vi "Read Intake Current.vi"(8 "Current":dbl, 9 "Proposed Power":dbl, 10 "Max Current":dbl, 11 "Current Trip Delay":dbl) -> (0 "Forward Tripped":bool, 1 "Backward Tripped":bool, 2 "Intake Current Trip State":T1, 3 "Actual Power":dbl, 4 "Current Over Max Current?":bool, 5 "Tripped?":bool)   [LabVIEW 2016]
uses:
  Common Code/Intake Trip States.ctl
  Common Code/Utilities/TimeManager.vi
  Common Code/Utilities/Change Detect.vi
  Common Code/Utilities/Change Detect Boolean.vi
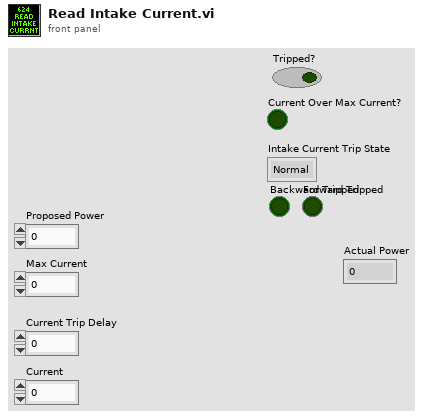
[diagram p1: front panel]
types:
  T1 = typedef "Intake Trip States.ctl" = enum16{"Normal", "Backward Tripped", "Forward Tripped"}
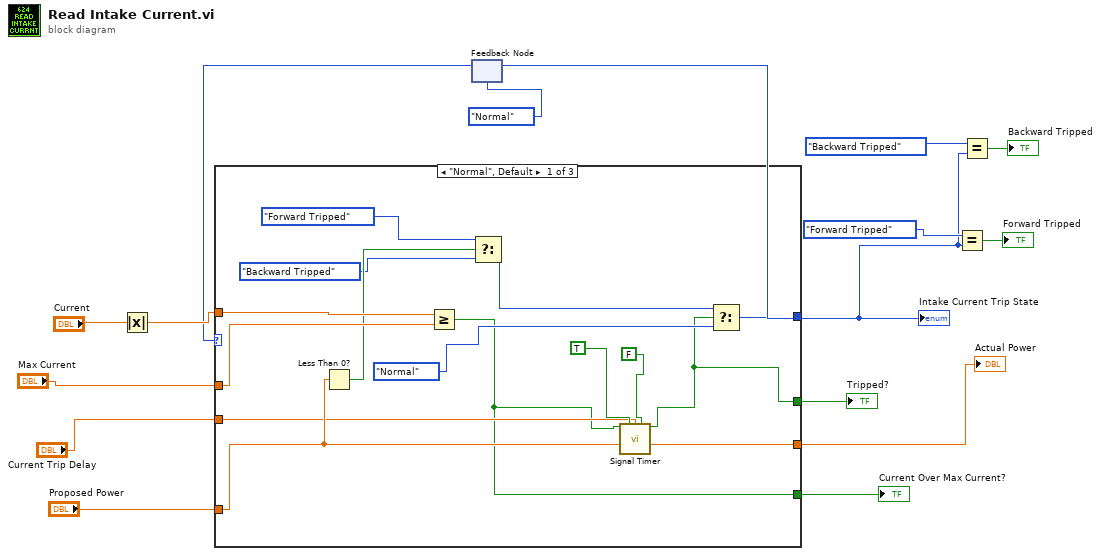
[diagram p0: block diagram]
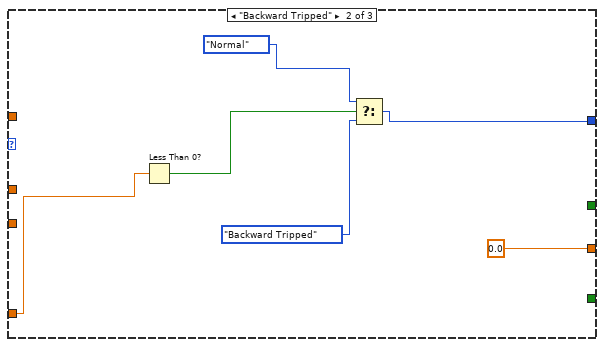
[diagram p2: hidden frame]
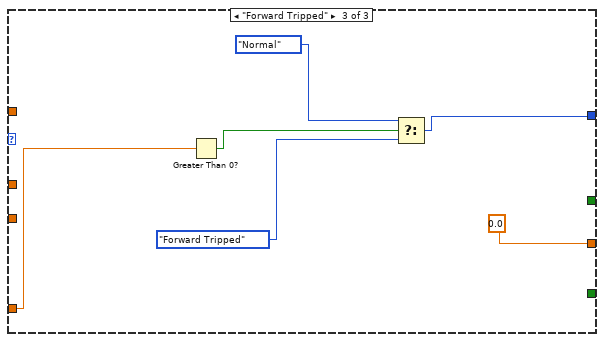
[diagram p3: hidden frame]
diagram:
  n1 = Absolute Value(x="Current") -> (abs(x)=w12:dbl)
  n2 = feedback #1(Intake_Trip_States."Normal" ("Intake Current Trip States")) -> (w3:T1)
  n3 = case shown="\"Normal\", Default" w3 {
    tunnel: "Proposed Power" -> [w25 w30 w40]
    tunnel: [w25 0.0 0.0] -> w15
    tunnel: "Max Current" -> [w28 _ _]
    tunnel: w12 -> [w29 _ _]
    tunnel: [w26 w35 w41] -> w4
    tunnel: "Current Trip Delay" -> [w19 _ _]
    tunnel: [w17 _ _] -> w2
    tunnel: [w16 _ _] -> w1
    frame "Normal", Default {
      n4 = Less Than 0?(x=w25) -> (x < 0?=w24:bool)
      n5 = Greater Or Equal?(x=w29, y=w28) -> (x >= y?=w16:bool)
      n6 = Select(t=Intake_Trip_States."Forward Tripped" ("Intake Current Trip States"), s=w24, f=Intake_Trip_States."Backward Tripped" ("Intake Current Trip States")) -> (s? t:f=w27:T1)
      n7 = call "Signal Timer.vi"("Input"=w16, "Edge"=TRUE, "Interval"=w19, "Pull"=FALSE) -> ("Filtered Output"=w17:bool)  [unwired: 11 in]
      n8 = Select(t=w27, s=w17, f=Intake_Trip_States."Normal" ("Intake Current Trip States")) -> (s? t:f=w26:T1)
    }
    frame "Backward Tripped" {
      n9 = Less Than 0?(x=w30) -> (x < 0?=w31:bool)
      n10 = Select(t=Intake_Trip_States."Normal" ("Intake Current Trip States"), s=w31, f=Intake_Trip_States."Backward Tripped" ("Intake Current Trip States")) -> (s? t:f=w35:T1)
    }
    frame "Forward Tripped" {
      n11 = Greater Than 0?(x=w40) -> (x > 0?=w39:bool)
      n12 = Select(t=Intake_Trip_States."Normal" ("Intake Current Trip States"), s=w39, f=Intake_Trip_States."Forward Tripped" ("Intake Current Trip States")) -> (s? t:f=w41:T1)
    }
  }
  "Actual Power" <- w15
  "Intake Current Trip State" <- w4
  "Tripped?" <- w2
  "Current Over Max Current?" <- w1
  n13 = feedback-in #1(w4) -> ()
  n14 = Equal?(x=Intake_Trip_States."Forward Tripped" ("Intake Current Trip States"), y=w4) -> (x = y?=→"Forward Tripped":bool)
  n15 = Equal?(x=Intake_Trip_States."Backward Tripped" ("Intake Current Trip States"), y=w4) -> (x = y?=→"Backward Tripped":bool)
